vi "DeviceRead.vi"(4 "error in (no error)":errorcluster, 6 "DeviceKey In":string, 7 "CmdLib In":refnum<k24>) -> (0 "error out":errorcluster, 1 "Response":string, 2 "DeviceKey Out":string, 3 "CmdLib Out":refnum<k24>)   [LabVIEW 2009]
uses:
  C:/Code/Apps/Utilities/Picomotor/PicomotorApp/Install/Samples/LabVIEW/Model 8743/LabVIEW 2009/CmdLib.dll
panel:
  in  "value":string
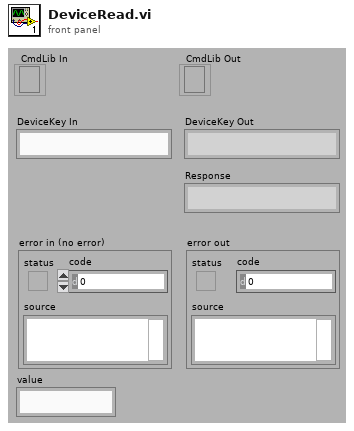
[diagram p1: front panel]
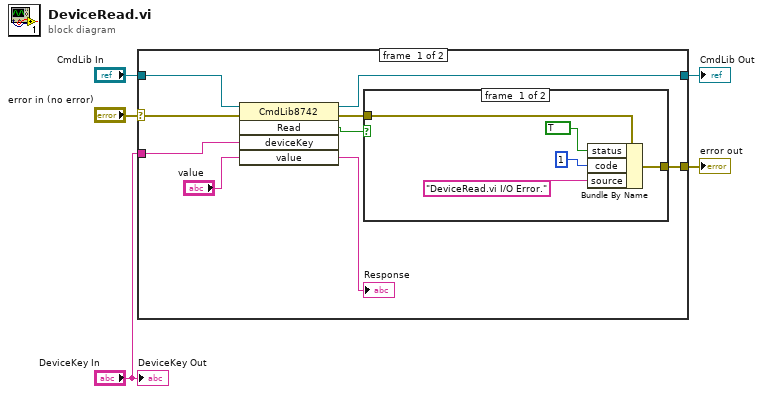
[diagram p0: block diagram]
diagram:
  n1 = case shown="No Error" "error in (no error)" {
    selector: "error in (no error)" -> [w11 w22]
    tunnel: "CmdLib In" -> [w14 w21]
    tunnel: [w13 w21] -> w4
    tunnel: "DeviceKey In" -> [w12 _]
    tunnel: [w8 w22] -> w1
    frame #0 {
      n2 = invoke class="CmdLib8742" method="Read"(reference=w14, error in=w11, "deviceKey"=w12, "value"="value") -> (reference out=w13:refnum<k24>, error out=w9:errorcluster, "Read"=w10:bool, "value"=→"Response":string)  [unwired: 1 in, 1 out]
      n3 = case shown="False" w10 {
        tunnel: w9 -> [w17 w20]
        tunnel: [w16 w20] -> w8
        frame #0 {
          n4 = Bundle By Name(cluster=w17, "status"=TRUE, "code"=1, "source"="DeviceRead.vi I/O Error.") -> (w16:errorcluster)
        }
        frame #1 {
        }
      }
    }
    frame #1 {
    }
  }
  "CmdLib Out" <- w4
  "error out" <- w1
  "DeviceKey Out" <- "DeviceKey In"
